vi "CuLab_Tensor_to_WF_Shifted.vi"(7 "dt":dbl, 11 "Y":sgl[](array[numeric])) -> (3 "WF":cluster{dbl, dbl, "Dest out":sgl[]})   [LabVIEW 2020]
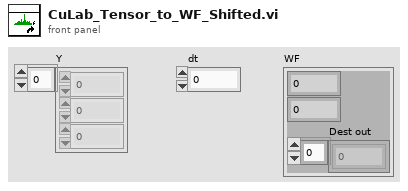
[diagram p1: front panel]
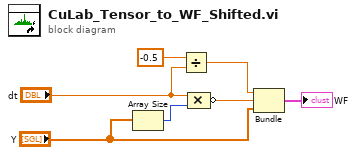
[diagram p0: block diagram]
diagram:
  n1 = Array Size(array="Y") -> (size(s)=w7:i32)
  n2 = Divide(x=-0.5 ("y"), y="dt") -> (x/y=w6:dbl)
  n3 = Compound Arithmetic op=MULTIPLY("dt", w7) -> (invert w5:dbl)
  n4 = Bundle(w6, w5, "Y"="Y") -> (→"WF":cluster{dbl, dbl, "Y":sgl[]})  [unwired: 1 in]
